vi "X10468 SLM Get Aberration Array.vi"(0 "Mode Amps":dbl[](array[numeric]), 7 "Zernike Modes":dbl[][][](array[numeric]), 11 "Error In":errorcluster) -> (8 "Aberration Array":dbl[][](array[numeric]), 15 "Error Out":errorcluster)   [LabVIEW 2018]
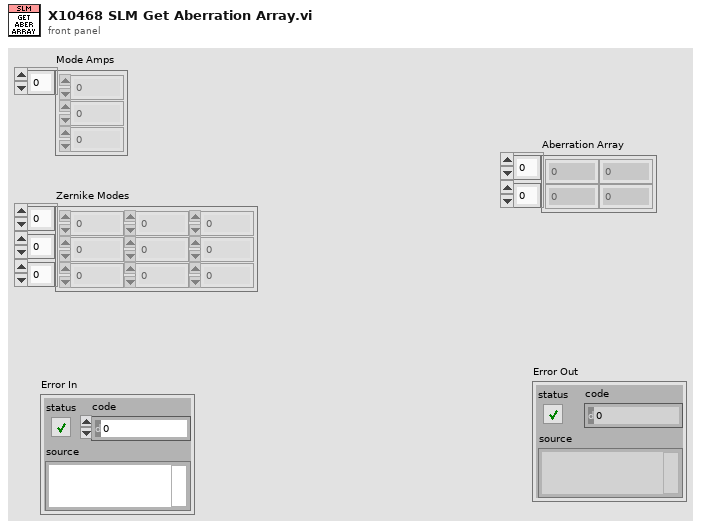
[diagram p1: front panel]
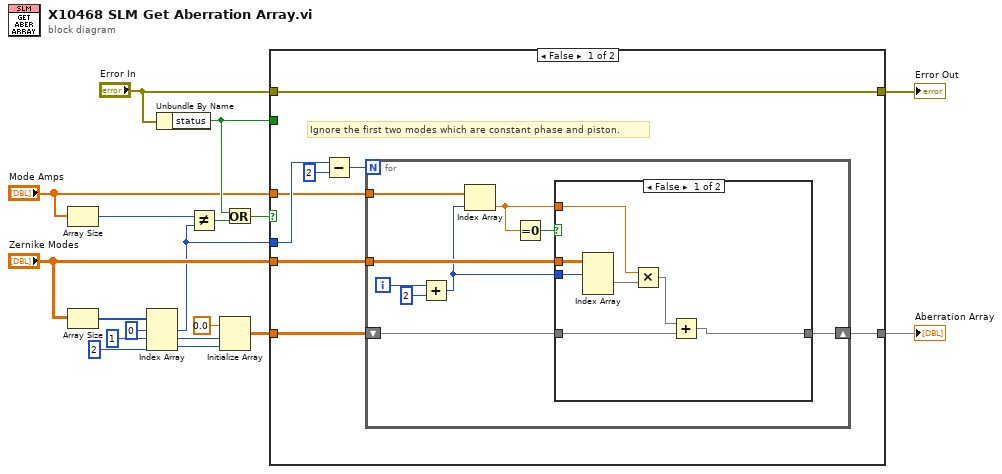
[diagram p0: block diagram]
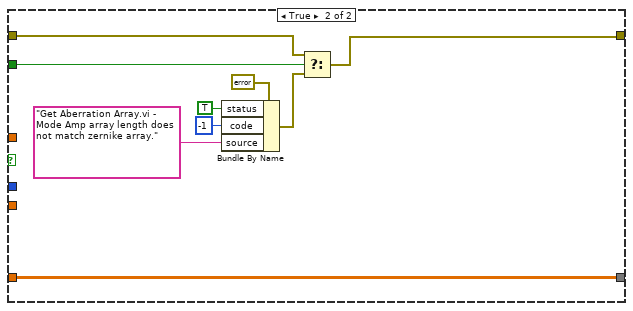
[diagram p3: hidden frame]
diagram:
  n1 = Array Size(array="Mode Amps") -> (size(s)=w14:i32)
  n2 = Array Size(array="Zernike Modes") -> (size(s)=w18:i32[])
  n3 = Index Array(array=w18, index #1=0 ("index"), index #2=1 ("index"), index #3=2 ("index")) -> (element #1=w8:i32, element #2=w4:i32, element #3=w3:i32)
  n4 = Unbundle By Name("Error In") -> ("status"=w11:bool)
  n5 = Not Equal?(x=w14, y=w8) -> (x != y?=w13:bool)
  n6 = Initialize Array(0.0 ("element"), w4, w3) -> (w2:dbl[][])
  n7 = Or(x=w11, y=w13) -> (x .or. y?=w12:bool)
  n8 = case shown="False" w12 {
    tunnel: w11 -> [_ w52]
    tunnel: "Mode Amps" -> [w21 _]
    tunnel: "Zernike Modes" -> [w25 _]
    tunnel: w8 -> [w24 _]
    tunnel: "Error In" -> [w26 w51]
    tunnel: [w26 w45] -> w6
    tunnel: w2 -> [w20 w44]
    tunnel: [w19 w44] -> w1
    frame False {
      # "Ignore the first two modes which are constant phase and piston."
      n9 = Subtract(x=w24, y=2) -> (x-y=w23:i32)
      n10 = for {
        N: w23 -> [_]
        shift-right: [w27] -> w19
        shift-left: w20 -> [w28]
        tunnel: w25 -> [w35]
        tunnel: w21 -> [w32]
        i -> [w34]
        n11 = Add(x=w34, y=2) -> (x+y=w31:i32)
        n12 = Index Array(array=w32, index=w31) -> (element=w29:dbl)
        n13 = Equal To 0?(x=w29) -> (x = 0?=w30:bool)
        n14 = case shown="False" w30 {
          tunnel: w35 -> [w42 _]
          tunnel: w31 -> [w41 _]
          tunnel: w29 -> [w39 _]
          tunnel: w28 -> [w38 w43]
          tunnel: [w36 w43] -> w27
          frame False {
            n15 = Index Array(array=w42, index (dim 0)=w41) -> (element=w40:dbl[][])  [unwired: 2 in]
            n16 = Multiply(x=w39, y=w40) -> (x*y=w37:dbl[][])
            n17 = Add(x=w37, y=w38) -> (x+y=w36:dbl[][])
          }
          frame True {
          }
        }
      }
    }
    frame True {
      n18 = Bundle By Name(cluster=errorcluster {"status"=FALSE, "code"=0, "source"=""} ("Error In"), "status"=TRUE, "code"=-1, "source"="Get Aberration Array.vi - Mode Amp array length does not match zernike array.") -> (w46:errorcluster)
      n19 = Select(t=w51, s=w52, f=w46) -> (s? t:f=w45:errorcluster)
    }
  }
  "Aberration Array" <- w1
  "Error Out" <- w6
